vi "解析串口信息.vi"(1 "16进制字符串":string) -> (0 "2进制字符串":string)   [LabVIEW 2014]
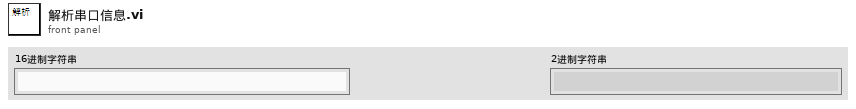
[diagram p1: front panel]
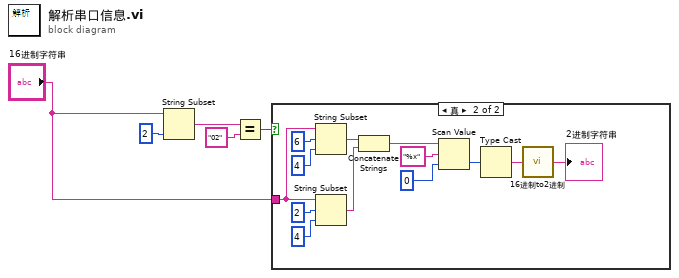
[diagram p0: block diagram]
diagram:
  n1 = String Subset(string="16进制字符串", length (rest)=2 ("长度（剩余）")) -> (substring=w4:string)  [unwired: 1 in]
  n2 = Equal?(x=w4, y="02") -> (x = y?=w2:bool)
  n3 = case shown="真" w2 {
    tunnel: "16进制字符串" -> [_ w14]
    frame False {
    }
    frame True {
      n4 = String Subset(string=w14, offset (0)=6 ("偏移量(0)"), length (rest)=4 ("长度（剩余）")) -> (substring=w13:string)
      n5 = String Subset(string=w14, offset (0)=2 ("偏移量(0)"), length (rest)=4 ("长度（剩余）")) -> (substring=w12:string)
      n6 = Concatenate Strings(w13, w12) -> (w11:string)
      n7 = Scan Value(string=w11, format string="%x", default (0 dbl)=0) -> (value=w8:i32)  [unwired: 1 out]
      n8 = Type Cast(x=w8) -> (*(type *) &x=w7:string)  [unwired: 1 in]
      n9 = call "16进制to2进制.vi"("16进制字符串"=w7) -> ("2进制字符串"=→"2进制字符串":string)
    }
  }
